vi "Set Matrix - stdin.vi"(7 "swap dimensions? (F)":bool, 8 "error in":errorcluster, 9 "value":dbl[][](array[numeric]), 10 "variable name":string, 11 "GOLPI ref. in":T1={"pipe handle"={"lv_proc.dll file path"=path "", "process instance handle"=[], "debug mode"=FALSE, "debug data"=[]}, "fast read timeout [ms]"=500, "fast read settle time [ms]"=10, "fast read to multiple [ms]"=1, "max elements per input line"=100, "slow read timeout [ms]"=5000, "stdin double format specifier"="%_16e", "max elements per stdout output column"=100}) -> (0 "error out":errorcluster, 3 "GOLPI ref. out":T1={"pipe handle"={"lv_proc.dll file path"=path "", "process instance handle"=[], "debug mode"=FALSE, "debug data"=[]}, "fast read timeout [ms]"=500, "fast read settle time [ms]"=10, "fast read to multiple [ms]"=1, "max elements per input line"=100, "slow read timeout [ms]"=5000, "stdin double format specifier"="%_16e", "max elements per stdout output column"=100})   [LabVIEW 2013, in "GOLPI library.lvlib"]
doc: "Writes double variable into GNU Octave by means of stdin. Supported are reals (doubles), complex and strings. Only one input can be nonempty array. Set terminal 'swap dimenstions?' if writing column vector."
uses:
  GOLPI library.lvlib
  Public/GOLPI reference Type Def.ctl
  LV Process source distribution/Pipe Handle.ctl
  LV Process source distribution/LV Process library.lvlib
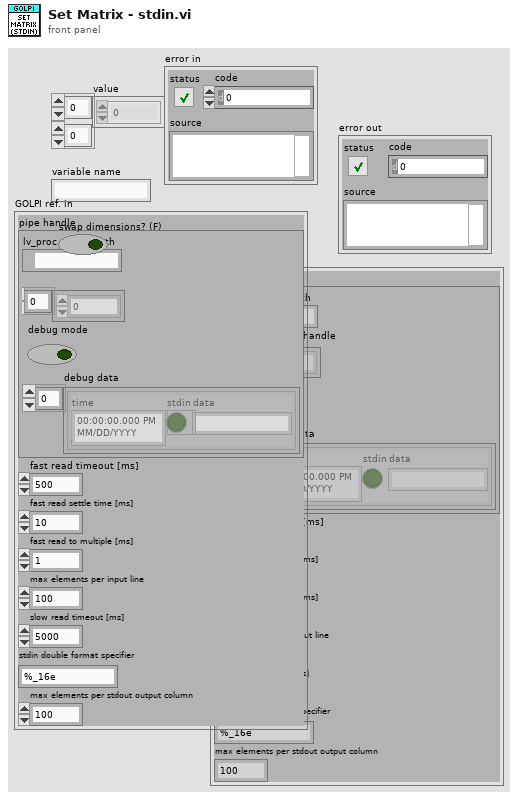
[diagram p1: front panel]
types:
  T1 = typedef "GOLPI library.lvlib/GOLPI reference Type Def.ctl" = cluster{"pipe handle":T2, "fast read timeout [ms]":u32, "fast read settle time [ms]":u32, "fast read to multiple [ms]":u32, "max elements per input line":u32, "slow read timeout [ms]":u32, "stdin double format specifier":string, "max elements per stdout output column":u32}
  T2 = typedef "LV Process library.lvlib/Pipe Handle.ctl" = cluster{"lv_proc.dll file path":path, "process instance handle":u32[], "debug mode":bool, "debug data":cluster{"time":timestamp, "stdin":bool, "data":string}[]}
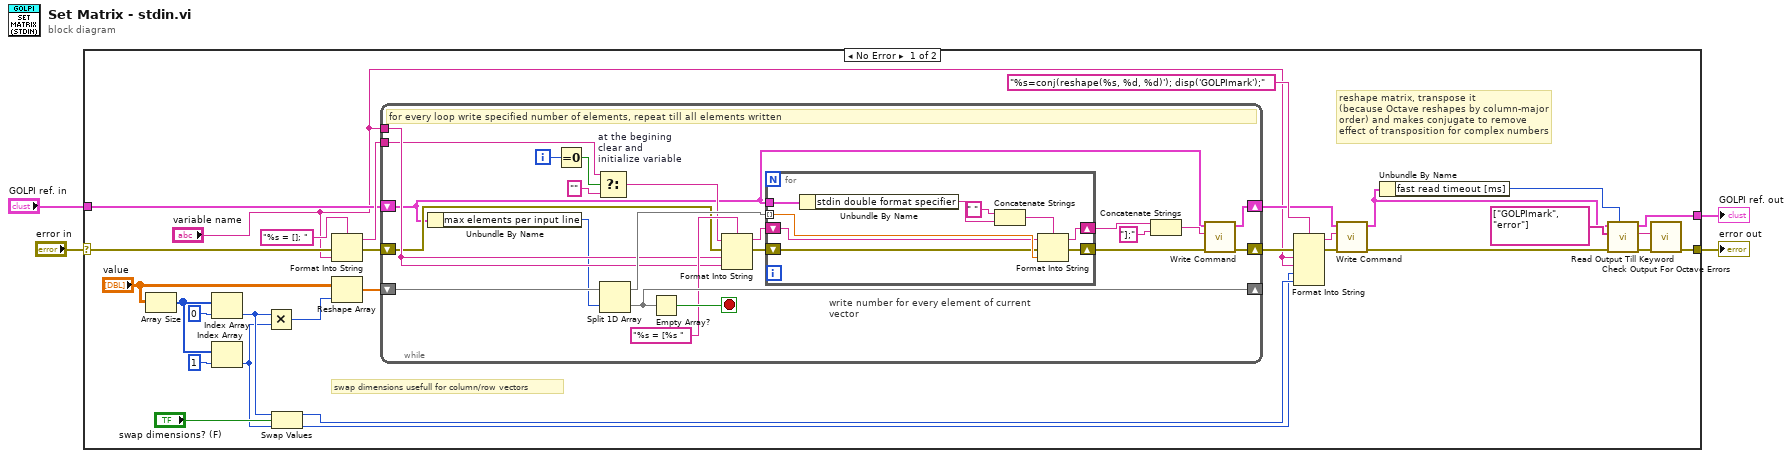
[diagram p0: block diagram]
diagram:
  n1 = case shown="No Error" "error in" {
    selector: "error in" -> [w16 w67]
    tunnel: [w17 w67] -> w4
    tunnel: "GOLPI ref. in" -> [w15 w66]
    tunnel: [w14 w66] -> w2
    frame No Error {
      # "swap dimensions usefull for column/row vectors"
      # "reshape matrix, transpose it\n(because Octave reshapes by column-major\norder) and makes conjugate to remove\neffect of transposition for complex numbers"
      n2 = Array Size(array="value") -> (size(s)=w30:i32[])
      n3 = Index Array(array=w30, index=0) -> (element=w9:i32)
      n4 = Index Array(array=w30, index=1) -> (element=w8:i32)
      n5 = Multiply(x=w9, y=w8) -> (x*y=w11:i32)
      n6 = Swap Values(12:w9, 13:"swap dimensions? (F)", 14:w8) -> (1:w6:i32, 3:w5:i32)
      n7 = Format Into String(format string="%s = []; ", error in=w16, "variable name") -> (resulting string=w25:string, error out=w33:errorcluster)  [unwired: 1 in]
      n8 = Reshape Array("value", w11) -> (w26:dbl[])
      n9 = while {
        shift-right: [w55] -> _
        shift-left: w26 -> [w56]
        tunnel: "variable name" -> [w48]
        shift-right: [w44] -> w34
        shift-left: w33 -> [w47]
        shift-right: [w43] -> w22
        shift-left: w15 -> [w35]
        tunnel: w25 -> [w39]
        i -> [w41]
        stop <- w54 stop-if-true
        # "for every loop write specified number of elements, repeat till all elements written"
        n10 = Unbundle By Name(w35) -> ("max elements per input line"=w36:u32)
        n11 = Equal To 0?(x=w41) -> (x = 0?=w40:bool)
        n12 = Select "at the begining\nclear and\ninitialize variable"(t=w39, s=w40, f="") -> (s? t:f=w38:string)
        n13 = Split 1D Array(array=w56, index=w36) -> (first subarray=w52:dbl[], second subarray=w55:dbl[])
        n14 = Empty Array?(array=w55) -> (empty?=w54:bool)
        n15 = Format Into String(format string="%s = [%s ", initial string=w38, error in=w47, w48, w48) -> (resulting string=w51:string, error out=w46:errorcluster)
        n16 = for "write number for every element of current vector" {
          tunnel: w52 -> [w65] mode=indexing
          shift-right: [w64] -> w50
          shift-left: w51 -> [w63]
          shift-right: [w61] -> w45
          shift-left: w46 -> [w62]
          tunnel: w35 -> [w59]
          n17 = Unbundle By Name(w59) -> ("stdin double format specifier"=w58:string)
          n18 = Concatenate Strings(" " ("string"), w58) -> (w57:string)
          n19 = Format Into String(format string=w57, initial string=w63, error in=w62, w65) -> (resulting string=w64:string, error out=w61:errorcluster)
        }
        n20 = Concatenate Strings(w50, "];" ("string")) -> (w42:string)
        n21 = call "Write Command.vi"("error in"=w45, "command"=w42, "GOLPI ref. in"=w35) -> ("error out"=w44:errorcluster, "GOLPI ref. out"=w43:T1)  [unwired: 7 in]
      }
      n22 = Format Into String(format string="%s=conj(reshape(%s, %d, %d)'); disp('GOLPImark');", error in=w34, "variable name", "variable name", w5, w6) -> (resulting string=w24:string, error out=w23:errorcluster)  [unwired: 1 in]
      n23 = call "Write Command.vi"("error in"=w23, "command"=w24, "GOLPI ref. in"=w22) -> ("error out"=w18:errorcluster, "GOLPI ref. out"=w13:T1)  [unwired: 7 in]
      n24 = Unbundle By Name(w13) -> ("fast read timeout [ms]"=w12:u32)
      n25 = call "Read Output Till Keyword.vi"("timeout [ms]"=w12, "error in"=w18, "keywords"=string[] ["GOLPImark", "error"], "GOLPI ref. in"=w13) -> ("error out"=w21:errorcluster, "read buffer"=w19:string, "GOLPI ref. out"=w14:T1)  [unwired: 4 in, 1 out]
      n26 = call "Check Output For Octave Errors.vi"("error in"=w21, "read buffer"=w19) -> ("error out"=w17:errorcluster)  [unwired: 9 in]
    }
    frame Error {
    }
  }
  "error out" <- w4
  "GOLPI ref. out" <- w2
